vi "Configure Measurements.vi"(6 "Measurement Type":enum16{"DCV", "ACV", "DCI", "ACI"}(ring), 8 "error in (no error)":errorcluster, 9 "Range":dbl, 10 "Scale":enum16{"1u", "1m", "1", "10", "100", "1k", "1M"}(ring), 11 "DMM in":refnum<class "DMM.lvclass">) -> (0 "error out":errorcluster, 3 "DMM out":refnum<class "DMM.lvclass">)   [LabVIEW 2020, in "DMM.lvclass"]
uses:
  DMM.lvclass
  DMM.lvclass/DMM.ctl
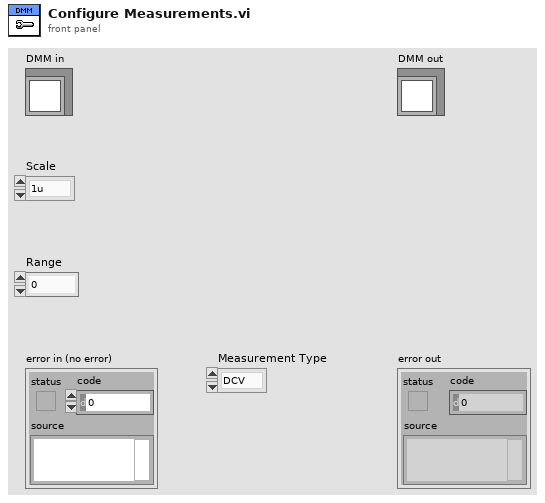
[diagram p1: front panel]
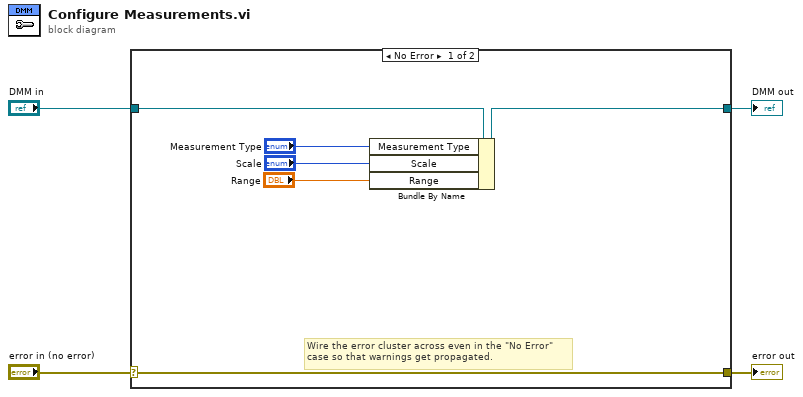
[diagram p0: block diagram]
diagram:
  n1 = case shown="No Error" "error in (no error)" {
    selector: "error in (no error)" -> [w9 w12]
    tunnel: [w9 w12] -> w3
    tunnel: [w8 w11] -> w1
    tunnel: "DMM in" -> [w10 w11]
    frame No Error {
      # "Wire the error cluster across even in the \"No Error\"\ncase so that warnings get propagated."
      n2 = Bundle By Name(cluster=w10, "Measurement Type"="Measurement Type", "Scale"="Scale", "Range"="Range") -> (w8:refnum<class "DMM.lvclass">)
    }
    frame Error {
    }
  }
  "error out" <- w3
  "DMM out" <- w1
